vi "Counter_SubVI.vi"(0 "s":bool) -> (7 "t":dbl)   [LabVIEW 2017]
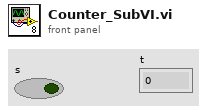
[diagram p1: front panel]
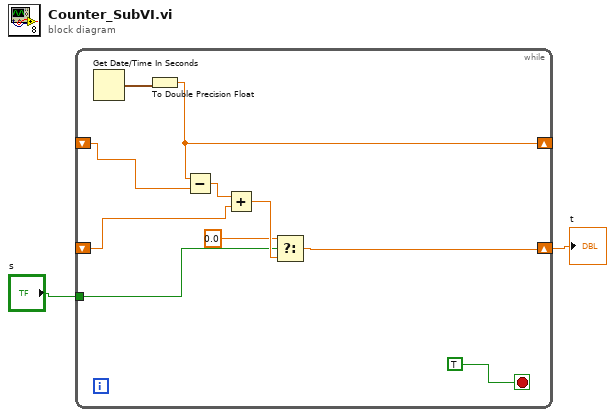
[diagram p0: block diagram]
diagram:
  n1 = while {
    shift-right: [w5] -> _
    shift-left: _ -> [w12]
    tunnel: "s" -> [w9]
    shift-right: [w8] -> w1
    shift-left: _ -> [w7]
    stop <- TRUE stop-if-true
    n2 = Get Date/Time In Seconds() -> (seconds since 1Jan1904=w6:timestamp)
    n3 = To Double Precision Float(number=w6) -> (double precision float=w5:dbl)
    n4 = Subtract(x=w5, y=w12) -> (x-y=w11:dbl)
    n5 = Add(x=w11, y=w7) -> (x+y=w10:dbl)
    n6 = Select(t=0.0, s=w9, f=w10) -> (s? t:f=w8:dbl)
  }
  "t" <- w1
